vi "Write Modbus Handle.vi"(8 "error in (no error)":errorcluster, 10 "Modbus Master":refnum<class "Modbus Master.lvclass">, 11 "Synchronization in":refnum<class "Synchronization.lvclass">) -> (0 "error out":errorcluster, 3 "Synchronization out":refnum<class "Synchronization.lvclass">)   [LabVIEW 2015, in "Synchronization Actor.lvlib" / "Synchronization.lvclass"]
uses:
  Synchronization.lvclass
  <vilib>/Modbus/master/Modbus Master.lvclass
  Synchronization.lvclass/Synchronization.ctl
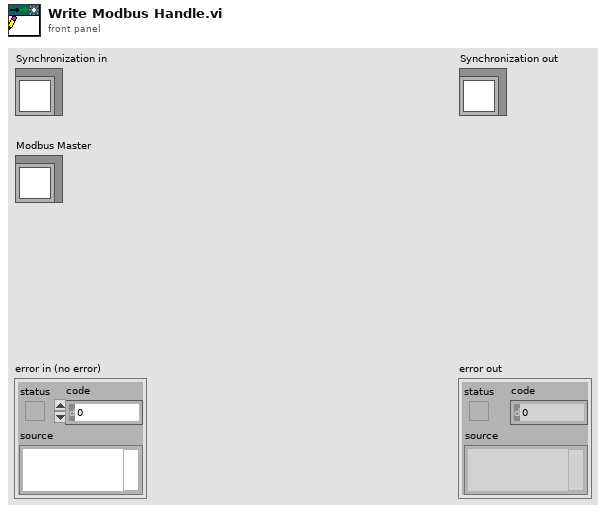
[diagram p1: front panel]
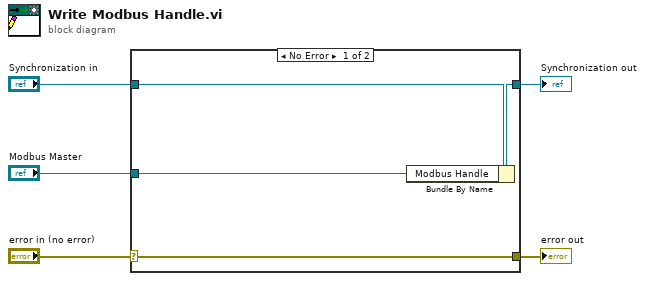
[diagram p0: block diagram]
diagram:
  n1 = case shown="No Error" "error in (no error)" {
    selector: "error in (no error)" -> [w9 w10]
    tunnel: [w9 w10] -> w4
    tunnel: [w7 w11] -> w2
    tunnel: "Synchronization in" -> [w8 w11]
    tunnel: "Modbus Master" -> [w6 _]
    frame No Error {
      n2 = Bundle By Name(cluster=w8, "Modbus Handle"=w6) -> (w7:refnum<class "Synchronization.lvclass">)
    }
    frame Error {
    }
  }
  "error out" <- w4
  "Synchronization out" <- w2
